vi "Configure Tone Operation.vi"(8 "error in (no error)":errorcluster, 9 "End Frequency Number (4)":i32=4, 10 "Tone Data":T1(array[cluster])=[{"Frequency (100 Hz)"=100.0, "Tone Start Condition (Triggered)"=1.0}] {"Tone Start Condition (Triggered)" items=["Triggered"=1.0, "Frequency Shift Key"=2.0, "Gated"=3.0]}, 11 "VISA resource name":refnum<visa-resource-name>) -> (0 "error out":errorcluster, 3 "VISA resource name out":refnum<visa-resource-name>)   [LabVIEW 2015, in "Fluke 28x Series.lvlib"]
doc: "Configures a set of up to 16 frequencies, under the control of the trigger input. The trigger input can be configured using the Configure Trigger Input VI. \n\nThe output (carrier waveform) is stepped through this list of frequencies consecutively."
uses:
  <instrlib>/Fluke 28x Series/Fluke 28x Series.lvlib
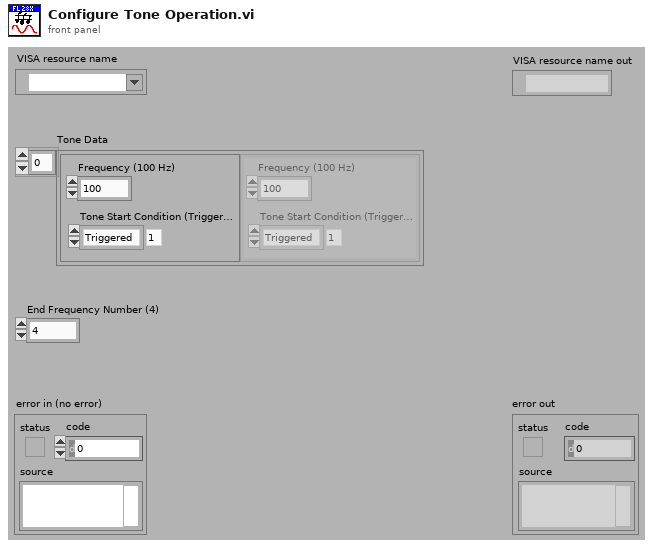
[diagram p1: front panel]
types:
  T1 = cluster{"Frequency (100 Hz)":dbl, "Tone Start Condition (Triggered)":dbl}[]
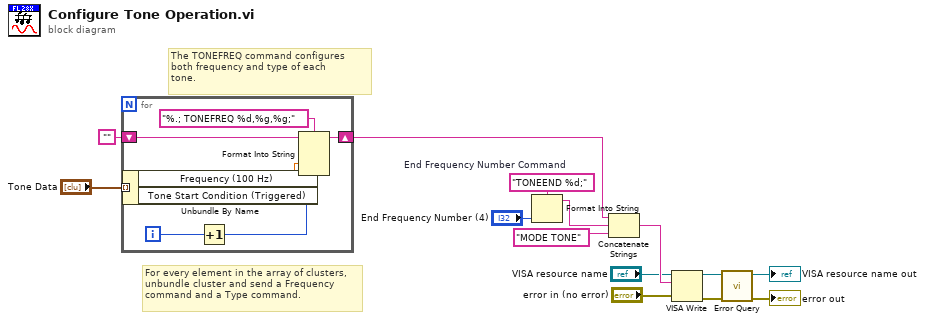
[diagram p0: block diagram]
diagram:
  w11 = "TONEEND %d;"  # End Frequency Number Command
  # "For every element in the array of clusters,\nunbundle cluster and send a Frequency \ncommand and a Type command."
  # "The TONEFREQ command configures\nboth frequency and type of each\ntone."
  n1 = for {
    tunnel: "Tone Data" -> [w21] mode=indexing
    shift-right: [w15] -> w6
    shift-left: "" ("Empty String Constant") -> [w16]
    i -> [w18]
    n2 = Unbundle By Name(w21) -> ("Frequency (100 Hz)"=w19:dbl, "Tone Start Condition (Triggered)"=w20:dbl)
    n3 = Increment(x=w18) -> (x+1=w17:i32)
    n4 = Format Into String(format string="%.; TONEFREQ %d,%g,%g;", initial string=w16, w17, w19, w20) -> (resulting string=w15:string)  [unwired: 1 in, 1 out]
  }
  n5 = Format Into String(format string=w11, "End Frequency Number (4)") -> (resulting string=w8:string)  [unwired: 2 in, 1 out]
  n6 = Concatenate Strings(w6, w8, "MODE TONE") -> (w5:string)
  n7 = VISA Write(VISA resource name="VISA resource name", write buffer=w5, error in (no error)="error in (no error)") -> (VISA resource name out=w13:refnum<visa-resource-name>, error out=w14:errorcluster)  [unwired: 1 out]
  n8 = call <instrlib>:"Error Query.vi"("error in (no error)"=w14, "VISA resource name"=w13) -> ("error out"=→"error out":errorcluster, "VISA resource name out"=→"VISA resource name out":refnum<visa-resource-name>)  [unwired: 6 in, 2 out]
